vi "Graphs 2.vi"() -> ()   [LabVIEW 2018]
panel:
  in  "Tab Control":enum32{"Page 1", "Page 2", "Page 3"}(tab)
  out "Waveform Chart":dbl(graph)
  out "Waveform Graph":dbl[](graph)
  out "Mixed Signal Graph":dbl[](graph)
  in  "Boolean":bool
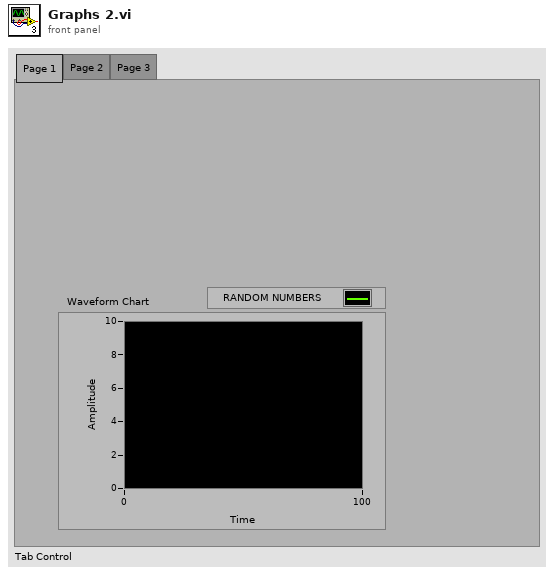
[diagram p1: front panel]
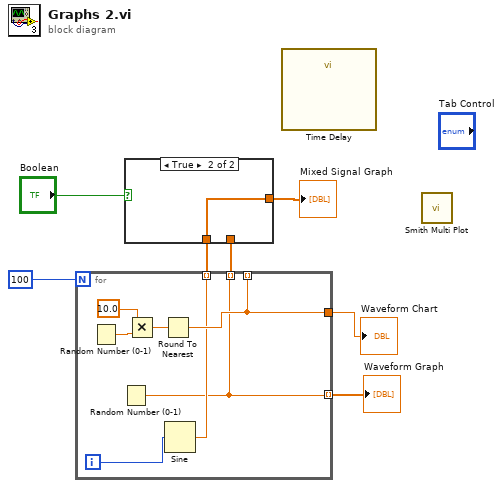
[diagram p0: block diagram]
diagram:
  n1 = for {
    N: 100 -> [_]
    tunnel: [w8] -> w7 mode=indexing
    tunnel: [w11] -> w5
    tunnel: [w11] -> _ mode=indexing
    tunnel: [w9] -> w2 mode=indexing
    tunnel: [w8] -> w1 mode=indexing
    i -> [w10]
    n2 = Random Number (0-1)() -> (number: 0 to 1=w14:dbl)
    n3 = Random Number (0-1)() -> (number: 0 to 1=w8:dbl)
    n4 = Multiply(x=10.0, y=w14) -> (x*y=w13:dbl)
    n5 = Round To Nearest(number=w13) -> (nearest integer value=w11:dbl)
    n6 = Sine(x=w10) -> (sin(x)=w9:dbl)
  }
  "Waveform Graph" <- w7
  "Waveform Chart" <- w5
  n7 = case shown="True" "Boolean" {
    tunnel: [w15 w16] -> w3
    tunnel: w2 -> [_ w16]
    tunnel: w1 -> [w15 _]
    frame False {
    }
    frame True {
    }
  }
  "Mixed Signal Graph" <- w3
  n8 = call "Time Delay"() -> ()  [unwired: 11 in, 1 out]
  n9 = call <vilib>:"Smith Multi Plot.vi"() -> ()  [unwired: 11 in, 1 out]
